vi "Pre Launch Init.vi"(11 "Cooler UI with Events in":refnum<class "Cooler UI with Events.lvclass">) -> (0 "error out":errorcluster, 3 "Cooler UI with Events out":refnum<class "Cooler UI with Events.lvclass">)   [LabVIEW 2012, in "Cooler UI.lvlib" / "Cooler UI with Events.lvclass"]
doc: "(<B>Filename</B>: Actor Framework.lvlib:Actor.lvclass:Pre Launch Init.vi)\n\nDefines behavior that occurs after the Launch Actor method is invoked but before the actor's Actor Core method begins running.\n\nThe Pre Launch Init method is guaranteed to finish before the Launch Actor method returns to its caller and before the actor itself receives any messages. Any references that the Pre Launch Init method obtains are guaranteed to have the same lifetime as the actor itself. Any errors that the Pre Launch Init method returns will abort the launch.\n\nBy default, this method does nothing. A descendant class may override it to define behavior."
uses:
  Cooler UI with Events.lvclass
  Status.ctl
  Cooler UI with Events.lvclass/Cooler UI with Events.ctl
  <vilib>/ActorFramework/Actor/Actor.lvclass
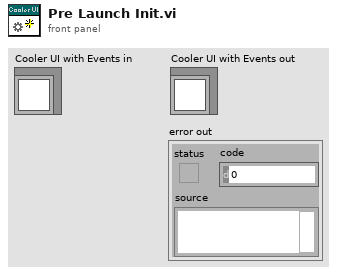
[diagram p1: front panel]
types:
  T1 = typedef "Cooler UI.lvlib/Cooler UI with Events.lvclass/Status.ctl" = cluster{"Fan A":cluster{"State":bool, "Fault":bool}, "Fan B":cluster{"State":bool, "Fault":bool}}
  T2 = cluster{"Fan Status":refnum<user-event>, "Temperature":refnum<user-event>, "Pump":refnum<user-event>}
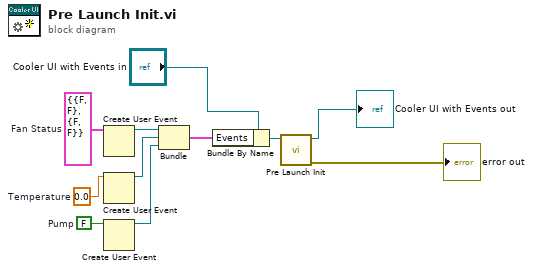
[diagram p0: block diagram]
diagram:
  w1 = FALSE  # Pump
  w2 = 0.0  # Temperature
  w3 = T1 {"Fan A"={"State"=FALSE, "Fault"=FALSE}, "Fan B"={"State"=FALSE, "Fault"=FALSE}}  # Fan Status
  n1 = Create User Event(user event datatype=w3) -> (user event=w6:refnum<user-event>)  [unwired: 1 in, 1 out]
  n2 = Create User Event(user event datatype=w2) -> (user event=w5:refnum<user-event>)  [unwired: 1 in, 1 out]
  n3 = Create User Event(user event datatype=w1) -> (user event=w4:refnum<user-event>)  [unwired: 1 in, 1 out]
  n4 = Bundle("Fan Status"=w6, "Temperature"=w5, "Pump"=w4) -> (w7:T2)  [unwired: 1 in]
  n5 = Bundle By Name(cluster="Cooler UI with Events in", "Events"=w7) -> (w8:refnum<class "Cooler UI with Events.lvclass">)
  n6 = call-parent "Pre Launch Init.vi"("Actor in"=w8) -> ("error out"=→"error out":errorcluster, "Actor out"=→"Cooler UI with Events out":refnum<class "Cooler UI with Events.lvclass">)  [unwired: 9 in]
